vi "Block Write Counter (SubVI).vi"(5 "Block Size":u16, 7 "Image Width":u16, 11 "Pixel Valid?":bool) -> (0 "Count":u16, 3 "Count End?":bool)   [LabVIEW 2015]
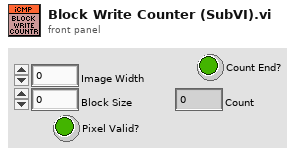
[diagram p1: front panel]
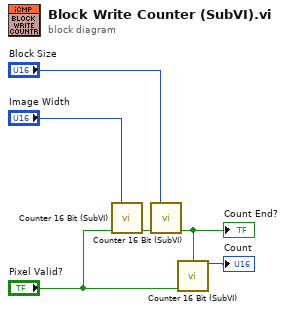
[diagram p0: block diagram]
diagram:
  n1 = call "Counter 16 Bit (SubVI).vi"("Max. Count"="Image Width", "Enable"="Pixel Valid?") -> ("Count End?"=w3:bool)  [unwired: 11 in, 2 out]
  n2 = call "Counter 16 Bit (SubVI).vi"("Max. Count"="Block Size", "Enable"=w3) -> ("Count End?"=w6:bool)  [unwired: 11 in, 2 out]
  "Count End?" <- w6
  n3 = call "Counter 16 Bit (SubVI).vi"("RESET"=w6, "Enable"="Pixel Valid?") -> ("Count"=→"Count":u16)  [unwired: 11 in, 2 out]
